vi "SVL Integration (frequency) (1 Ch).vi"(0 "spectrum":cluster{"f0":dbl, "df":dbl, "magnitude":dbl[]} {"magnitude" format="%.2f"; "df" format="%.2f"; "f0" format="%.2f"}, 1 "integration type":T7(ring)=enum."double integration", 4 "spectrum info in":T1={"channel name"="", "description"="", "x-axis units"=0, "spectral info"={"spectrum type"=enum."Power [Magnitude^2]", "linear/dB"=enum."linear", "window"=0, "window size"=0, "FFT size"=0}, "engineering units"=0, "custom label"="", "dB reference [EU]"=0.0, "peak units"=enum."rms", "weighting filter"=0, "spectral density?"=FALSE, "unit label"="", "spectrum skewed?"=FALSE, "complimentary spectrum units"=enum."none"} {"x-axis units" items=["Time (s)"=0, "Frequency-CB (Hz)"=1, "Frequency-CPB (Hz)"=1248, "Frequency-Arbitrary (Hz)"=2357, "Quefrency (s)"=2, "Revolutions (rev)"=3, "Order"=4, "Speed (RPM)"=11, "Speed (rad/s)"=21, "Index"=65535]; "weighting filter" items=["Linear", "A-weighting", "B-weighting", "C-weighting", "ITU-R 468-4", "Dolby", "CCITT", "C-message", "Wb", "Wc", "Wd", "We", "Wf", "Wh", "Wj", "Wk", "Wm", "AES17 20 kHz lowpass", "AES17 40 kHz lowpass", "AES17 20 kHz highpass", "AES17 40 kHz highpass"]; "dB reference [EU]" format="%.2f"; "engineering units" items=["custom..."=0, "V"=1, "A"=21, "C"=30, "pC"=31, "s"=32, "-"=29, "Pa"=2, "N"=20, "g"=3, "m/s^2"=4, "m/s"=5, "m"=6, "mm/s"=12, "mm"=13, "micron/s"=14, "micron"=15, "in/s^2"=7, "in/s"=8, "in"=9, "mil/s"=10, "mil"=11, "rad/s^2"=16, "rad/s"=17, "rad"=18, "deg/s^2"=26, "deg/s"=27, "deg"=28, "RPM"=22, "cycle/s^2"=23, "Hz"=24, "cycle"=25, "strain"=19]; "spectral info"."window" items=["None "=0, "Hanning"=1, "Hamming"=2, "Blackman-Harris"=3, "Exact Blackman"=4, "Blackman"=5, "Flat Top"=6, "4 Term B-Harris "=7, "7 Term B-Harris"=8, "Low Sidelobe"=9, "Force - Exponential"=10, "Gaussian"=62]}, 5 "error in (no error)":errorcluster, 6 "length units":i32(ring) items=["no change"=-1, "m"=0, "mm"=2, "microns"=3, "in"=1, "mils"=5]) -> (14 "integrated spectrum":cluster{"f0":dbl, "df":dbl, "magnitude":dbl[]} {"magnitude" format="%.2f"; "df" format="%.2f"; "f0" format="%.2f"}, 15 "unit label":string, 18 "spectrum info out":T1={"channel name"="", "description"="", "x-axis units"=0, "spectral info"={"spectrum type"=enum."Power [Magnitude^2]", "linear/dB"=enum."linear", "window"=0, "window size"=0, "FFT size"=0}, "engineering units"=0, "custom label"="", "dB reference [EU]"=0.0, "peak units"=enum."rms", "weighting filter"=0, "spectral density?"=FALSE, "unit label"="", "spectrum skewed?"=FALSE, "complimentary spectrum units"=enum."none"} {"x-axis units" items=["Time (s)"=0, "Frequency-CB (Hz)"=1, "Frequency-CPB (Hz)"=1248, "Frequency-Arbitrary (Hz)"=2357, "Quefrency (s)"=2, "Revolutions (rev)"=3, "Order"=4, "Speed (RPM)"=11, "Speed (rad/s)"=21, "Index"=65535]; "weighting filter" items=["Linear", "A-weighting", "B-weighting", "C-weighting", "ITU-R 468-4", "Dolby", "CCITT", "C-message", "Wb", "Wc", "Wd", "We", "Wf", "Wh", "Wj", "Wk", "Wm", "AES17 20 kHz lowpass", "AES17 40 kHz lowpass", "AES17 20 kHz highpass", "AES17 40 kHz highpass"]; "dB reference [EU]" format="%.2f"; "engineering units" items=["custom..."=0, "V"=1, "A"=21, "C"=30, "pC"=31, "s"=32, "-"=29, "Pa"=2, "N"=20, "g"=3, "m/s^2"=4, "m/s"=5, "m"=6, "mm/s"=12, "mm"=13, "micron/s"=14, "micron"=15, "in/s^2"=7, "in/s"=8, "in"=9, "mil/s"=10, "mil"=11, "rad/s^2"=16, "rad/s"=17, "rad"=18, "deg/s^2"=26, "deg/s"=27, "deg"=28, "RPM"=22, "cycle/s^2"=23, "Hz"=24, "cycle"=25, "strain"=19]; "spectral info"."window" items=["None "=0, "Hanning"=1, "Hamming"=2, "Blackman-Harris"=3, "Exact Blackman"=4, "Blackman"=5, "Flat Top"=6, "4 Term B-Harris "=7, "7 Term B-Harris"=8, "Low Sidelobe"=9, "Force - Exponential"=10, "Gaussian"=62]}, 19 "error out":errorcluster)   [LabVIEW 2017, in "SoundVib_Integration.lvlib"]
doc: "Converts acceleration to velocity or displacement using a frequency spectrum as the input. Wire data to the <B>spectrum</B> input to determine the polymorphic instance to use or manually select the instance."
uses:
  <vilib>/addons/Sound and Vibration/svt_Integration/SoundVib_Integration.lvlib
  <vilib>/addons/_NISVFA/_Shared subVIs/Controls/svc_Spectrum Info.ctl
  <vilib>/addons/_NISVFA/_Shared subVIs/Controls/svc_X-Axis Units.ctl
  <vilib>/addons/_NISVFA/_Shared subVIs/Controls/svc_Spectrum Type.ctl
  <vilib>/addons/_NISVFA/_Shared subVIs/Controls/svc_Engineering Units Text Ring.ctl
  <vilib>/addons/_NISVFA/_Shared subVIs/Controls/svc_Weighting Filter Text Ring.ctl
  <vilib>/addons/_NISVFA/_Shared subVIs/Controls/svc_Complimentary Spectrum Units.ctl
  <vilib>/addons/_NISVFA/_Shared subVIs/Common/svc_Create X Array from x0 dx and length.vi
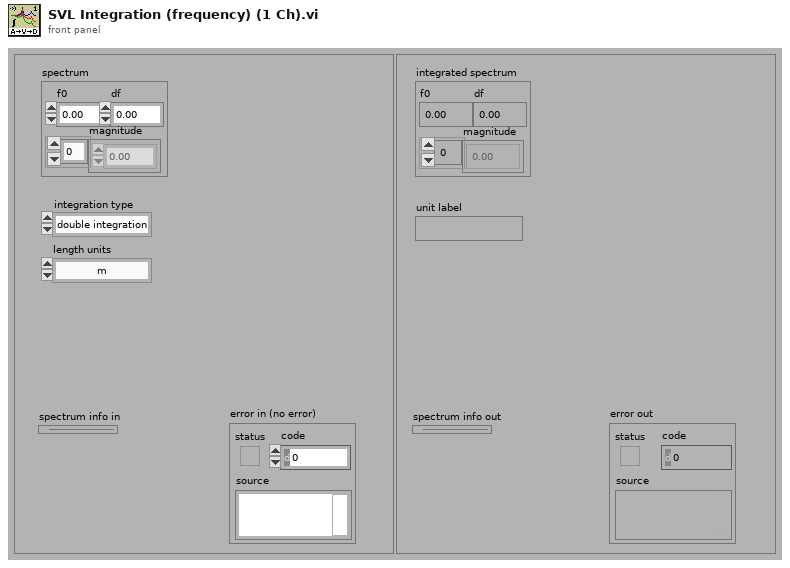
[diagram p1: front panel]
types:
  T1 = typedef "svc_Spectrum Info.ctl" = cluster{"channel name":string, "description":string, "x-axis units":T2, "spectral info":cluster{"spectrum type":T3, "linear/dB":enum16{"linear", "dB"}, "window":u16, "window size":i32, "FFT size":i32}, "engineering units":T4, "custom label":string, "dB reference [EU]":dbl, "peak units":enum16{"rms", "peak", "peak-peak"}, "weighting filter":T5, "spectral density?":bool, "unit label":string, "spectrum skewed?":bool, "complimentary spectrum units":T6}
  T2 = typedef "svc_X-Axis Units.ctl" = u16
  T3 = typedef "svc_Spectrum Type.ctl" = enum16{"FFT Spectrum [complex]", "Amplitude [Magnitude]", "Power [Magnitude^2]", "Cross Spectrum [complex]", "Frequency Response [Complex]"}
  T4 = typedef "svc_Engineering Units Text Ring.ctl" = u16
  T5 = typedef "svc_Weighting Filter Text Ring.ctl" = u16
  T6 = typedef "svc_Complimentary Spectrum Units.ctl" = enum16{"none", "radians", "degrees", "cycles", "imaginary"}
  T7 = enum16{"single integration", "double integration"}
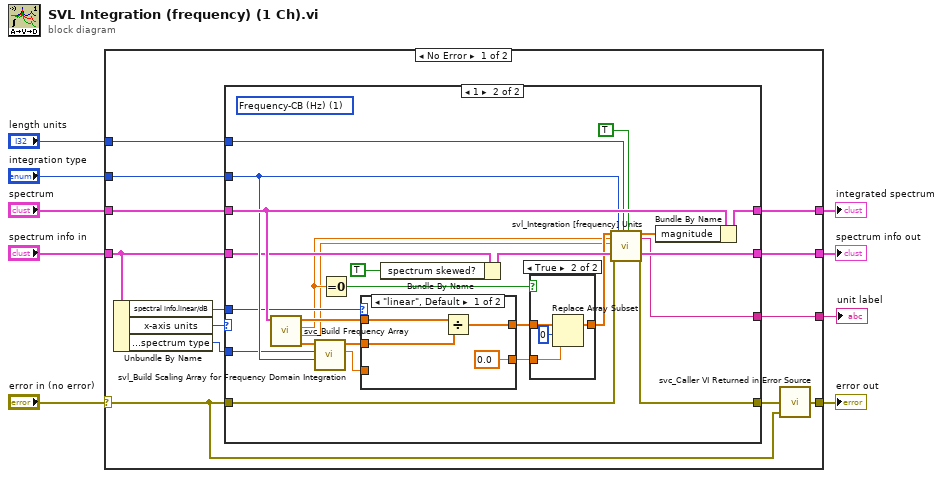
[diagram p0: block diagram]
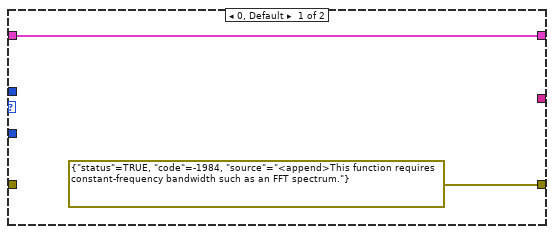
[diagram p2: hidden frame]
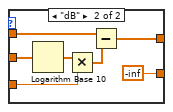
[diagram p4: hidden frame]
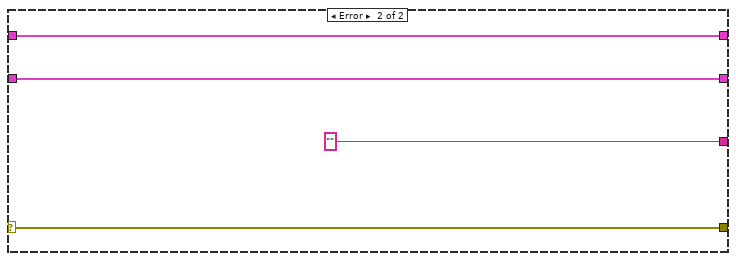
[diagram p5: hidden frame]
diagram:
  n1 = case shown="No Error" "error in (no error)" {
    selector: "error in (no error)" -> [w11 w68]
    tunnel: [w22 w69] -> w9
    tunnel: "spectrum" -> [w21 w69]
    tunnel: "integration type" -> [w20 _]
    tunnel: "spectrum info in" -> [w17 w67]
    tunnel: [w12 w68] -> w4
    tunnel: [w16 w67] -> w3
    tunnel: "length units" -> [w15 _]
    tunnel: [w14 "" ("unit label")] -> w1
    frame No Error {
      n2 = Unbundle By Name(w17) -> ("spectral info.linear/dB"=w19:enum16{"linear", "dB"}, "x-axis units"=w10:T2, "spectral info.spectrum type"=w13:T3)
      n3 = case shown="1" w10 {
        tunnel: [_ w49] -> w22
        tunnel: w21 -> [_ w48]
        tunnel: w20 -> [_ w47]
        tunnel: w19 -> [_ w46]
        tunnel: [errorcluster {"status"=TRUE, "code"=-1984, "source"="<append>This function requires constant-frequency bandwidth such as an FFT spectrum."} ("error out") w45] -> w18
        tunnel: w17 -> [w24 w44]
        tunnel: [w24 w43] -> w16
        tunnel: w15 -> [_ w42]
        tunnel: [_ w41] -> w14
        tunnel: w13 -> [_ w40]
        tunnel: w11 -> [_ w39]
        frame 0, Default {
        }
        frame 1 {
          (unwired) T2 1 items=["Time (s)"=0, "Frequency-CB (Hz)"=1, "Frequency-CPB (Hz)"=1248, "Frequency-Arbitrary (Hz)"=2357, "Quefrency (s)"=2, "Revolutions (rev)"=3, "Order"=4, "Speed (RPM)"=11, "Speed (rad/s)"=21, "Critical Band"=31, "Critical Band Rate (Bark)"=32, "None"=98, "Index"=65535] ("x-axis units")
          n4 = call <vilib>:"svc_Build Frequency Array.vi"("spectrum"=w48) -> ("frequency array [Hz]"=w29:dbl[], "df [Hz]"=w26:dbl, "f0"=w27:dbl, "magnitude"=w30:dbl[])  [unwired: 7 in]
          n5 = call <vilib>:"svl_Build Scaling Array for Frequency Domain Integration.vi"("integration type"=w47, "spectrum type"=w40, "frequency array [Hz]"=w29) -> ("dB multiplier"=w32:dbl, "scaling array"=w31:dbl[])  [unwired: 7 in]
          n6 = Equal To 0?(x=w27) -> (x = 0?=w37:bool)
          n7 = case shown="\"linear\", Default" w46 {
            tunnel: w30 -> [w58 w62]
            tunnel: [w56 w60] -> w38
            tunnel: w31 -> [w57 w65]
            tunnel: w32 -> [_ w63]
            tunnel: [0.0 ("New Element/Subarray") -inf] -> w36
            frame "linear", Default {
              n8 = Divide(x=w58, y=w57) -> (x/y=w56:dbl[])
            }
            frame "dB" {
              n9 = Logarithm Base 10(1:w65) -> (0:w64:dbl[])
              n10 = Multiply(x=w64, y=w63) -> (x*y=w61:dbl[])
              n11 = Subtract(x=w62, y=w61) -> (x-y=w60:dbl[])
            }
          }
          n12 = Bundle By Name(cluster=w44, "spectrum skewed?"=TRUE) -> (w34:T1)
          n13 = case shown="True" w37 {
            tunnel: w38 -> [w50 w53]
            tunnel: [w50 w52] -> w28
            tunnel: w36 -> [_ w51]
            frame False {
            }
            frame True {
              n14 = Replace Array Subset(array=w53, new element=w51, index=0 ("Index")) -> (w52:dbl[])
            }
          }
          n15 = call <vilib>:"svl_Integration [frequency] Units.vi"("spectrum"=w28, "f0"=w27, "df [Hz]"=w26, "spectrum info in"=w34, "error in"=w39, "integration type"=w47, "desired base units for length"=w42, "automatically convert peak units"=TRUE ("convert displacement to peak units")) -> ("spectrum"=w25:dbl[], "unit label"=w41:string, "spectrum info out"=w43:T1, "error out"=w45:errorcluster)  [unwired: 8 in]
          n16 = Bundle By Name(cluster=w48, "magnitude"=w25) -> (w49:cluster{"f0":dbl, "df":dbl, "magnitude":dbl[]})
        }
      }
      n17 = call <vilib>:"svc_Caller VI Returned in Error Source.vi"("warning input to caller"=w11, "error in (no error)"=w18) -> ("error out"=w12:errorcluster)  [unwired: 3 in]
    }
    frame Error {
    }
  }
  "integrated spectrum" <- w9
  "error out" <- w4
  "spectrum info out" <- w3
  "unit label" <- w1
